vi "Find Nearest Color.vi"(10 "Color":u32(colorbox), 11 "Color Palette":u32[](array[numeric])) -> (2 "Indexed Color":u32(colorbox), 3 "Index":i32)   [LabVIEW 2020, in "G-Image.lvlib"]
doc: "Find the closest match in Color Palette of the RGB color. Index is the index of the closest color match in the Color Palette array, and Indexed Color is the value of that color."
uses:
  G-Image.lvlib
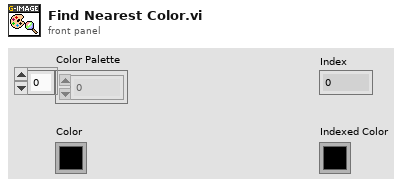
[diagram p1: front panel]
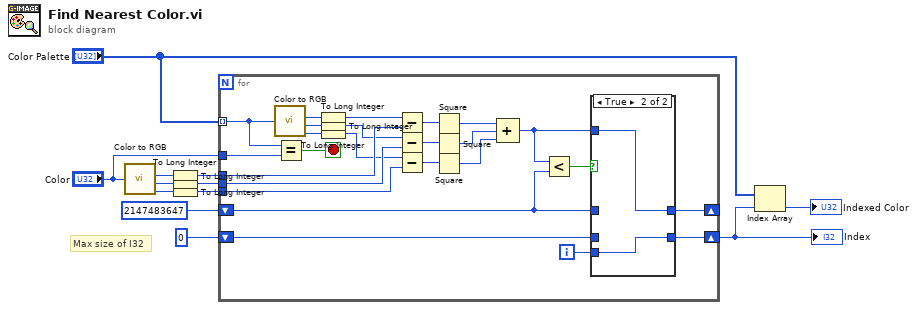
[diagram p0: block diagram]
diagram:
  # "Max size of I32"
  n1 = call <vilib>:"Color to RGB.vi"("Color"="Color") -> ("R"=w12:u8, "G"=w11:u8, "B"=w10:u8)  [unwired: 1 out]
  n2 = To Long Integer(number=w12) -> (32bit integer=w9:i32)
  n3 = To Long Integer(number=w11) -> (32bit integer=w8:i32)
  n4 = To Long Integer(number=w10) -> (32bit integer=w7:i32)
  n5 = for {
    shift-right: [w26] -> _
    shift-left: 2147483647 -> [w24]
    tunnel: w9 -> [w36]
    tunnel: w8 -> [w34]
    tunnel: w7 -> [w32]
    tunnel: "Color Palette" -> [w15] mode=indexing
    shift-right: [w23] -> w3
    shift-left: 0 -> [w27]
    tunnel: "Color" -> [w14]
    i -> [w22]
    stop <- w13 stop-if-true
    n6 = call <vilib>:"Color to RGB.vi"("Color"=w15) -> ("R"=w37:u8, "G"=w35:u8, "B"=w33:u8)  [unwired: 1 out]
    n7 = Equal?(x=w15, y=w14) -> (x = y?=w13:bool)
    n8 = To Long Integer(number=w37) -> (32bit integer=w31:i32)
    n9 = To Long Integer(number=w35) -> (32bit integer=w30:i32)
    n10 = To Long Integer(number=w33) -> (32bit integer=w29:i32)
    n11 = Subtract(x=w31, y=w36) -> (x-y=w21:i32)
    n12 = Subtract(x=w30, y=w34) -> (x-y=w20:i32)
    n13 = Subtract(x=w29, y=w32) -> (x-y=w19:i32)
    n14 = Square(x=w21) -> (x^2=w18:i32)
    n15 = Square(x=w20) -> (x^2=w17:i32)
    n16 = Square(x=w19) -> (x^2=w16:i32)
    n17 = Compound Arithmetic op=ADD(w18, w17, w16) -> (w25:i32)
    n18 = Less?(x=w25, y=w24) -> (x < y?=w28:bool)
    n19 = case shown="True" w28 {
      tunnel: w27 -> [w38 _]
      tunnel: [w39 w41] -> w26
      tunnel: w25 -> [_ w41]
      tunnel: w24 -> [w39 _]
      tunnel: [w38 w40] -> w23
      tunnel: w22 -> [_ w40]
      frame False {
      }
      frame True {
      }
    }
  }
  "Index" <- w3
  n20 = Index Array(array="Color Palette", index=w3) -> (element=→"Indexed Color":u32)
